vi "Write Pulse Width.vi"(8 "error in":errorcluster, 10 "Pulse Width":dbl, 11 "3300 in":refnum<class "3300.lvclass">) -> (0 "error out":errorcluster, 3 "3300 out":refnum<class "3300.lvclass">)   [LabVIEW 2019, in "3300.lvlib" / "3300.lvclass"]
uses:
  Library/3300.lvclass
  builds/Instruments/Electronic Load.lvlibp/Library/Electronic Load.lvclass
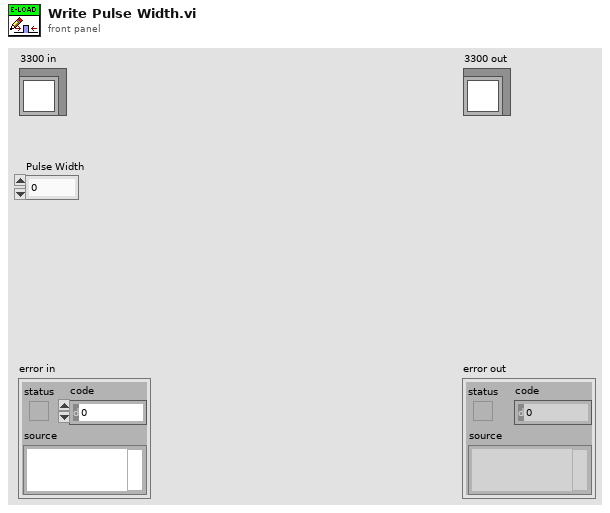
[diagram p1: front panel]
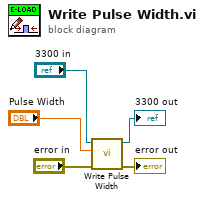
[diagram p0: block diagram]
diagram:
  n1 = call-parent "Write Pulse Width.vi"("error in"="error in", "Pulse Width"="Pulse Width", "Electronic Load in"="3300 in") -> ("error out"=→"error out":errorcluster, "Electronic Load out"=→"3300 out":refnum<class "3300.lvclass">)  [unwired: 7 in]
